vi "RF to dB.vi"(8 "Error In":errorcluster, 9 "RF":dbl[][](array[numeric])) -> (0 "Error Out":errorcluster, 1 "dB":dbl[][](array[numeric]))   [LabVIEW 2019]
uses:
  <vilib>/Analysis/NI_AALPro.lvlib
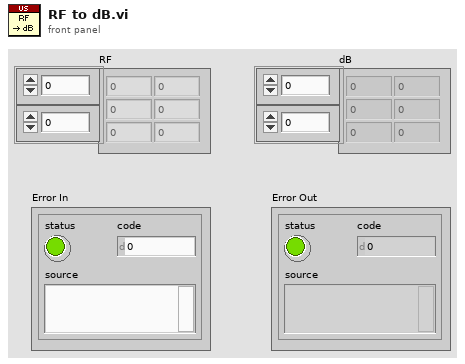
[diagram p1: front panel]
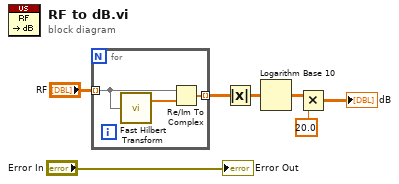
[diagram p0: block diagram]
diagram:
  n1 = for {
    tunnel: "RF" -> [w9] mode=indexing
    tunnel: [w8] -> w1 mode=indexing
    n2 = call <vilib>:"Fast Hilbert Transform.vi"("X"=w9) -> ("Hilbert{X}"=w10:dbl[])  [unwired: 1 out]
    n3 = Re/Im To Complex(1:w10, 2:w9) -> (0:w8:cdb[])
  }
  n4 = Absolute Value(x=w1) -> (abs(x)=w4:dbl[][])
  n5 = Logarithm Base 10(1:w4) -> (0:w5:dbl[][])
  n6 = Multiply(x=w5, y=20.0) -> (x*y=→"dB":dbl[][])
  "Error Out" <- "Error In"
